vi "Pipe Var Intf - Read Variable Data.vi"(7 "timeout [ms]":i32=3000, 8 "error in (no error)":errorcluster, 11 "pipe handle":i32) -> (0 "error out":errorcluster, 1 "data type":T1=enum."String", 2 "data out":u8[](array[numeric]), 3 "pipe handle out":i32, 4 "rows":i32, 6 "columns":i32)   [LabVIEW 2020, in "GOLPI library.lvlib"]
doc: "Tries to write variable binary data with header for the Pipe Variable Interface."
uses:
  GOLPI library.lvlib
  Pipe Var Intf - Data Type.ctl
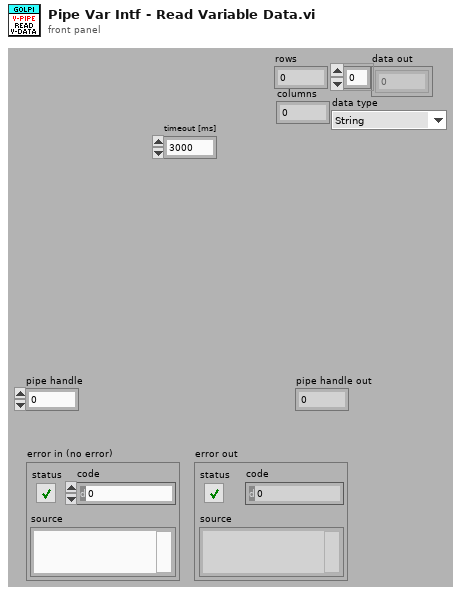
[diagram p1: front panel]
types:
  T1 = typedef "GOLPI library.lvlib/Pipe Var Intf - Data Type.ctl" = enum16{"error", "String", "int8", "uint8", "int16", "uint16", "int32", "uint32", "double", "cplx double", "single", "cplx single"}
  T2 = enum16{"big-endian, network order", "native, host order", "little-endian"}
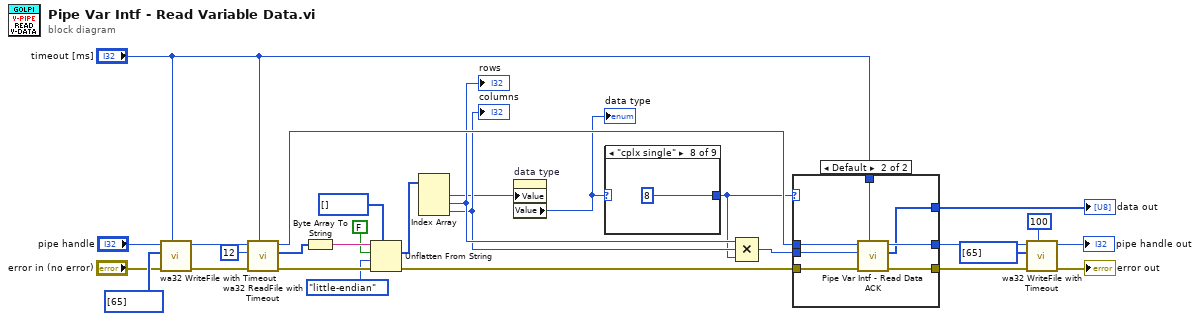
[diagram p0: block diagram]
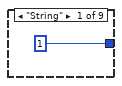
[diagram p3: hidden frame]
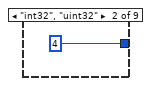
[diagram p4: hidden frame]
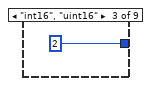
[diagram p5: hidden frame]
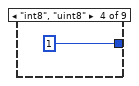
[diagram p6: hidden frame]
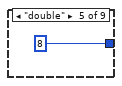
[diagram p7: hidden frame]
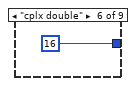
[diagram p8: hidden frame]
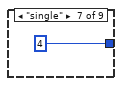
[diagram p9: hidden frame]
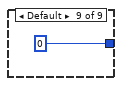
[diagram p10: hidden frame]
diagram:
  n1 = call "wa32 WriteFile with Timeout.vi"("timeout [ms]"="timeout [ms]", "error in (no error)"="error in (no error)", "data"=u8[] [65], "pipe handle"="pipe handle") -> ("error out"=w9:errorcluster, "pipe handle out"=w8:i32)  [unwired: 5 in, 1 out]
  n2 = call "wa32 ReadFile with Timeout.vi"("timeout [ms]"="timeout [ms]", "error in (no error)"=w9, "read count (0: all)"=12, "pipe handle"=w8) -> ("error out"=w28:errorcluster, "data out"=w27:u8[], "pipe handle out"=w20:i32)  [unwired: 4 in, 1 out]
  n3 = Byte Array To String(unsigned byte array=w27) -> (string=w26:string)
  n4 = Unflatten From String(type=i32[] [], binary string=w26, data includes array or string size? (T)=FALSE, byte order (0:big-endian, network order)=T2."little-endian", error in (no error)=w28) -> (value=w22:i32[], error out=w21:errorcluster)  [unwired: 1 out]
  n5 = Index Array(array=w22) -> (element #1=w4:i32, element #2=w19:i32, element #3=w18:i32)  [unwired: 3 in]
  "rows" <- w19
  "columns" <- w18
  n6 = property on="data type" class="Enum (strict)"("Value"=w4) -> ("Value"=w3:T1)  [unwired: 2 in, 2 out]
  "data type" <- w3
  n7 = case shown="\"cplx single\"" w3 {
    tunnel: [1 4 2 1 8 16 4 8 0] -> w16
    frame "String" {
    }
    frame "int32", "uint32" {
    }
    frame "int16", "uint16" {
    }
    frame "int8", "uint8" {
    }
    frame "double" {
    }
    frame "cplx double" {
    }
    frame "single" {
    }
    frame "cplx single" {
    }
    frame Default {
    }
  }
  n8 = Compound Arithmetic op=MULTIPLY(w19, w18, w16) -> (w17:i32)
  n9 = case shown="Default" w16 {
    tunnel: w21 -> [w40 w47]
    tunnel: w20 -> [w39 w46]
    tunnel: w17 -> [_ w45]
    tunnel: "timeout [ms]" -> [_ w44]
    tunnel: [w40 w43] -> w14
    tunnel: [w39 w42] -> w13
    tunnel: [_ w41] -> w15
    frame 0 {
    }
    frame Default {
      n10 = call "Pipe Var Intf - Read Data ACK.vi"("timeout [ms]"=w44, "error in (no error)"=w47, "read count"=w45, "pipe handle"=w46) -> ("error out"=w43:errorcluster, "data out"=w41:u8[], "pipe handle out"=w42:i32)  [unwired: 4 in, 1 out]
    }
  }
  "data out" <- w15
  n11 = call "wa32 WriteFile with Timeout.vi"("timeout [ms]"=100, "error in (no error)"=w14, "data"=u8[] [65], "pipe handle"=w13) -> ("error out"=→"error out":errorcluster, "pipe handle out"=→"pipe handle out":i32)  [unwired: 5 in, 1 out]
